vi "CmdWriter.vi"() -> ()   [LabVIEW 2020]
doc: "Copyright © 2008 - 2024 VI Technologies B.V. \nALL RIGHTS RESERVED"
uses:
  SuperNS/SuperNS.lvclass
  MsgData/MsgData.lvclass
panel:
  out "error out":errorcluster
  in  "My Name":string="CmdWriter"
  in  "Reader URL":string="//localhost/CmdReader"
  in  "Send":bool
  in  "Msg":string
  # "Copyright (c) 2024, VI Technologies B.V.\nAll rights reserved.\n\nRedistribution and use in source and binary forms, with or without modification, are permitted provided that \nthe following conditions are met:\n\n * Redistributions of source code must retain the above copyright notice, this list of conditions and the \nfollowing disclaimer.\n * Redistributions in binary form must reproduce the above copyright notice, this list of conditions and the \nfollowing disclaimer in the documentation and/or other materials provided with the distribution.\n * Neither the name of VI Technologies B.V. nor the names of its contributors may be used to endorse or \npromote products derived from this software without specific prior written permission.\n\nTHIS SOFTWARE IS PROVIDED BY THE COPYRIGHT HOLDERS AND CONTRIBUTORS \"AS IS\" AND ANY EXPRESS OR \nIMPLIED WARRANTIES, INCLUDING, BUT NOT LIMITED TO, THE IMPLIED WARRANTIES OF MERCHANTABILITY \nAND FITNESS FOR A PARTICULAR PURPOSE ARE DISCLAIMED. IN NO EVENT SHALL THE COPYRIGHT OWNER OR \nCONTRIBUTORS BE LIABLE FOR ANY DIRECT, INDIRECT, INCIDENTAL, SPECIAL, EXEMPLARY, OR CONSEQUENTIAL \nDAMAGES (INCLUDING, BUT NOT LIMITED TO, PROCUREMENT OF SUBSTITUTE GOODS OR SERVICES; LOSS OF \nUSE, DATA, OR PROFITS; OR BUSINESS INTERRUPTION) HOWEVER CAUSED AND ON ANY THEORY OF LIABILITY, \nWHETHER IN CONTRACT, STRICT LIABILITY, OR TORT (INCLUDING NEGLIGENCE OR OTHERWISE) ARISING IN ANY \nWAY OUT OF THE USE OF THIS SOFTWARE, EVEN IF ADVISED OF THE POSSIBILITY OF SUCH DAMAGE.\n\nFor more information, please visit https://www.vi-tech.nl or contact us at info@vi-tech.nl"
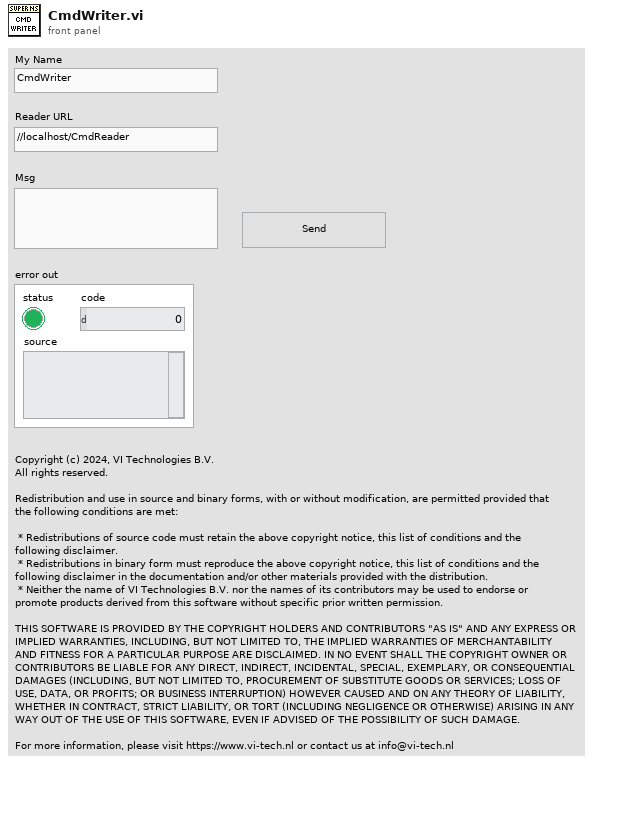
[diagram p1: front panel]
types:
  T1 = enum16{"None (High througput mode)", "All Elements Read From Stream", "All Elements Available for Reading"}
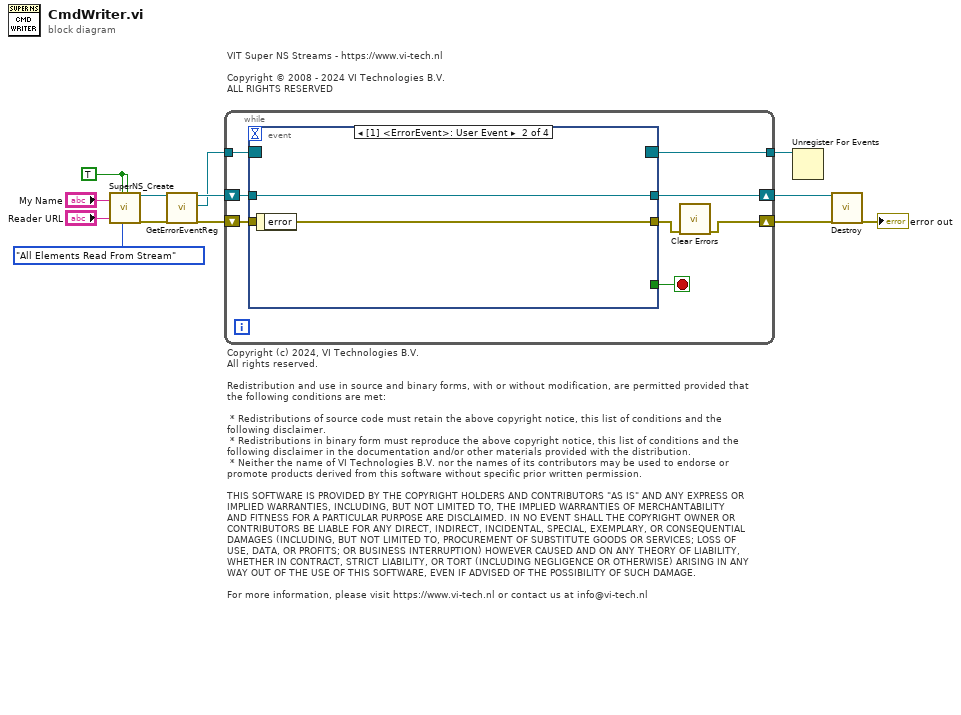
[diagram p0: block diagram]
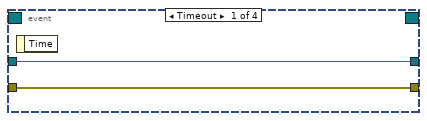
[diagram p2: hidden frame]
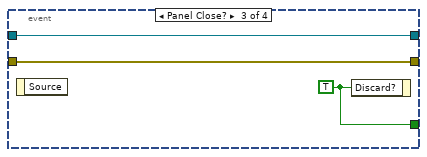
[diagram p3: hidden frame]
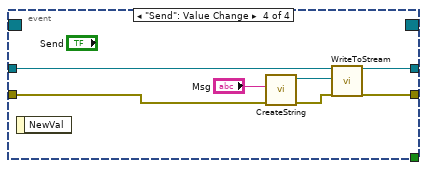
[diagram p4: hidden frame]
diagram:
  w7 = TRUE ("Writer")
  # "VIT Super NS Streams - https://www.vi-tech.nl\n\nCopyright © 2008 - 2024 VI Technologies B.V. \nALL RIGHTS RESERVED"
  # "Copyright (c) 2024, VI Technologies B.V.\nAll rights reserved.\n\nRedistribution and use in source and binary forms, with or without modification, are permitted provided that \nthe following conditions are met:\n\n * Redistributions of source code must retain the above copyright notice, this list of conditions and the \nfollowing disclaimer.\n * Redistributions in binary form must reproduce the above copyright notice, this list of conditions and the \nfollowing disclaimer in the documentation and/or other materials provided with the distribution.\n * Neither the name of VI Technologies B.V. nor the names of its contributors may be used to endorse or \npromote products derived from this software without specific prior written permission.\n\nTHIS SOFTWARE IS PROVIDED BY THE COPYRIGHT HOLDERS AND CONTRIBUTORS \"AS IS\" AND ANY EXPRESS OR \nIMPLIED WARRANTIES, INCLUDING, BUT NOT LIMITED TO, THE IMPLIED WARRANTIES OF MERCHANTABILITY \nAND FITNESS FOR A PARTICULAR PURPOSE ARE DISCLAIMED. IN NO EVENT SHALL THE COPYRIGHT OWNER OR \nCONTRIBUTORS BE LIABLE FOR ANY DIRECT, INDIRECT, INCIDENTAL, SPECIAL, EXEMPLARY, OR CONSEQUENTIAL \nDAMAGES (INCLUDING, BUT NOT LIMITED TO, PROCUREMENT OF SUBSTITUTE GOODS OR SERVICES; LOSS OF \nUSE, DATA, OR PROFITS; OR BUSINESS INTERRUPTION) HOWEVER CAUSED AND ON ANY THEORY OF LIABILITY, \nWHETHER IN CONTRACT, STRICT LIABILITY, OR TORT (INCLUDING NEGLIGENCE OR OTHERWISE) ARISING IN ANY \nWAY OUT OF THE USE OF THIS SOFTWARE, EVEN IF ADVISED OF THE POSSIBILITY OF SUCH DAMAGE.\n\nFor more information, please visit https://www.vi-tech.nl or contact us at info@vi-tech.nl"
  n1 = call "SuperNS_Create.vi"("NSName"="My Name", "RemoteEP_URL"="Reader URL", "Writer (F: Reader)"=w7, "Low latency mode"=T1."All Elements Read From Stream", "OpenProcessWindow"=w7) -> ("SuperNS Reference"=w5:refnum<class "SuperNS.lvclass">, "error out"=w12:errorcluster)  [unwired: 13 in]
  n2 = call-dynamic "GetErrorEventReg.vi"("reference in"=w5, "error in"=w12) -> ("reference out"=w4:refnum<class "SuperNS.lvclass">, "ErrorEventReg"=w3:refnum<event-registration>, "error out"=w6:errorcluster)  [unwired: 15 in]
  n3 = while {
    shift-right: [w16] -> w10
    shift-left: w4 -> [w17]
    shift-right: [w20] -> w13
    shift-left: w6 -> [w21]
    tunnel: w3 -> [w15]
    tunnel: [w14] -> w2
    stop <- w18 stop-if-true
    n4 = event shown="[1] <ErrorEvent>: User Event" {
      selector: w15 -> [_ _ _ _]
      dyn-events: [_ _ _ _] -> w14
      timeout: _ -> [_ _ _ _]
      tunnel: [_ _ w28 _] -> w18
      tunnel: [w22 w25 w27 w33] -> w16
      tunnel: w17 -> [w22 w25 w27 w34]
      tunnel: w21 -> [w23 _ w26 w29]
      tunnel: [w23 w24 w26 w35] -> w19
      event Timeout {
        n5 = event-data() -> ()  [unwired: 1 in, 1 out]
      }
      event User Event {
        n6 = event-data() -> ("error"=w24:errorcluster)  [unwired: 1 in]
      }
      event Panel Close? {
        w28 = TRUE ("Discard?")
        n7 = event-data() -> ()  [unwired: 1 in, 1 out]
        n8 = event-data("Discard?"=w28) -> ()  [unwired: 1 in, 1 out]
      }
      event "Send": Value Change {
        n9 = event-data() -> ()  [unwired: 1 in, 1 out]
        n10 = call "CreateString.vi"("error in"=w29, "String"="Msg") -> ("error out"=w30:errorcluster, "MsgData out"=w31:refnum<class "MsgData.lvclass">)  [unwired: 8 in]
        n11 = call-dynamic "WriteToStream.vi"("reference in"=w34, "LabVIEW Object"=w31, "error in"=w30) -> ("reference out"=w33:refnum<class "SuperNS.lvclass">, "error out"=w35:errorcluster)  [unwired: 14 in, 1 out]
      }
    }
    n12 = call <vilib>:"Clear Errors.vi"("error in (no error)"=w19) -> ("error out"=w20:errorcluster)  [unwired: 5 in, 1 out]
  }
  n13 = Unregister For Events(event registration refnum=w2) -> ()  [unwired: 1 in, 1 out]
  n14 = call-dynamic "Destroy.vi"("reference in"=w10, "error in (no error)"=w13) -> ("error out"=→"error out":errorcluster)  [unwired: 16 in, 1 out]
